vi "HEWH_Inficon.vi"(8 "error in":errorcluster, 11 "Message Queues out":T1) -> (0 "error out":errorcluster)   [LabVIEW 2023]
uses:
  Tenney/support/Message Queue/All Message Queues.ctl
  Tenney/support/Message Queue/Message Cluster.ctl
  <vilib>/NI/Modbus Library/API/Master/Modbus Master.lvclass
  Drivers/Inficon Fusion Micro GC/Type Definitions/Inficon Data.ctl
  <vilib>/NI/Modbus Library/API/Wrapper/Create TCP Master.vi
  FVIR and LDO/support/Message Queue/Enqueue Message (Single).vi
  FVIR and LDO/support/Message Queue/Message Queue.lvlib
  <vilib>/NI/Modbus Library/API/Wrapper/API Main.lvlib
  Tenney/support/Message Queue/Tenney Message Queue.lvlib
panel:
  out "Debug List":string[](array[string])
  in  "Debug":bool
  out "Loop Count":i32
  # "Need to send this value from the main program"
  # "NG Inficon: 192.168.1.32\nLP Inficon: 192.168.1.33"
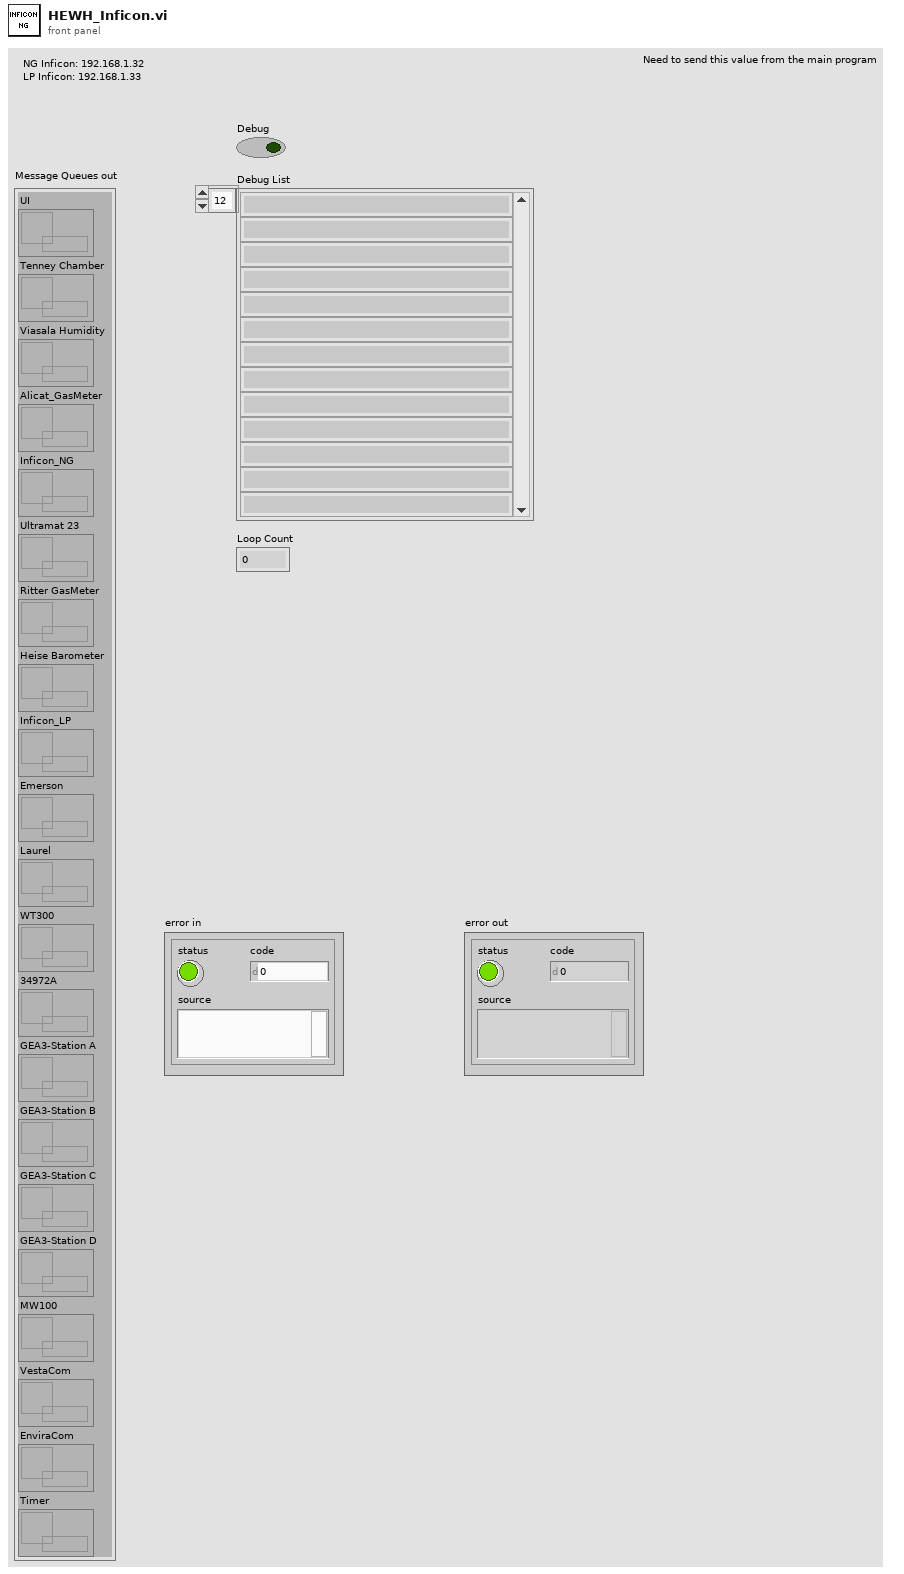
[diagram p1: front panel]
types:
  T1 = typedef "Tenney Message Queue.lvlib/All Message Queues.ctl" = cluster{"UI":refnum<queue>, "Tenney Chamber":refnum<queue>, "Viasala Humidity":refnum<queue>, "Alicat_GasMeter":refnum<queue>, "Inficon_NG":refnum<queue>, "Ultramat 23":refnum<queue>, "Ritter GasMeter":refnum<queue>, "Heise Barometer":refnum<queue>, "Inficon_LP":refnum<queue>, "Emerson":refnum<queue>, "Laurel":refnum<queue>, "WT300":refnum<queue>, "34972A":refnum<queue>, "GEA3-Station A":refnum<queue>, "GEA3-Station B":refnum<queue>, "GEA3-Station C":refnum<queue>, "GEA3-Station D":refnum<queue>, "MW100":refnum<queue>, "VestaCom":refnum<queue>, "EnviraCom":refnum<queue>, "Timer":refnum<queue>}
  T2 = typedef "Inficon Data.ctl" = cluster{"Gross Heating Value, Vol (Real, Dry)":dbl, "Nitrogen Component Normalized Mole % (Dry)":dbl, "Methane Component Normalized Mole % (Dry)":dbl, "Carbon Dioxide Component Normalized Mole % (Dry)":dbl, "Ethane Component Normalized Mole % (Dry)":dbl, "Propane Component Normalized Mole % (Dry)":dbl, "i-Pentane Component Normalized Mole % (Dry)":dbl, "i-Butane Component Normalized Mole % (Dry)":dbl, "n-Butane Component Normalized Mole % (Dry)":dbl, "n-Pentane Component Normalized Mole % (Dry)":dbl, "Hexane Component Normalized Mole % (Dry)":dbl, "Heptane Component Normalized Mole % (Dry)":dbl, "Gross Wobbe Index, Real(Dry)":dbl, "Relative Density, Real(Dry)":dbl, "Propylene Component Normalized Mole % (Dry)":dbl, "C4 Olefins Component Normalized Mole % (Dry)":dbl, "Water Component Normalized Mole % (Dry)":dbl, "Gross Heating Value, Vol (Real, Sat)":dbl, "Natural Gas Data":string[][], "Propane Data":string[][]}
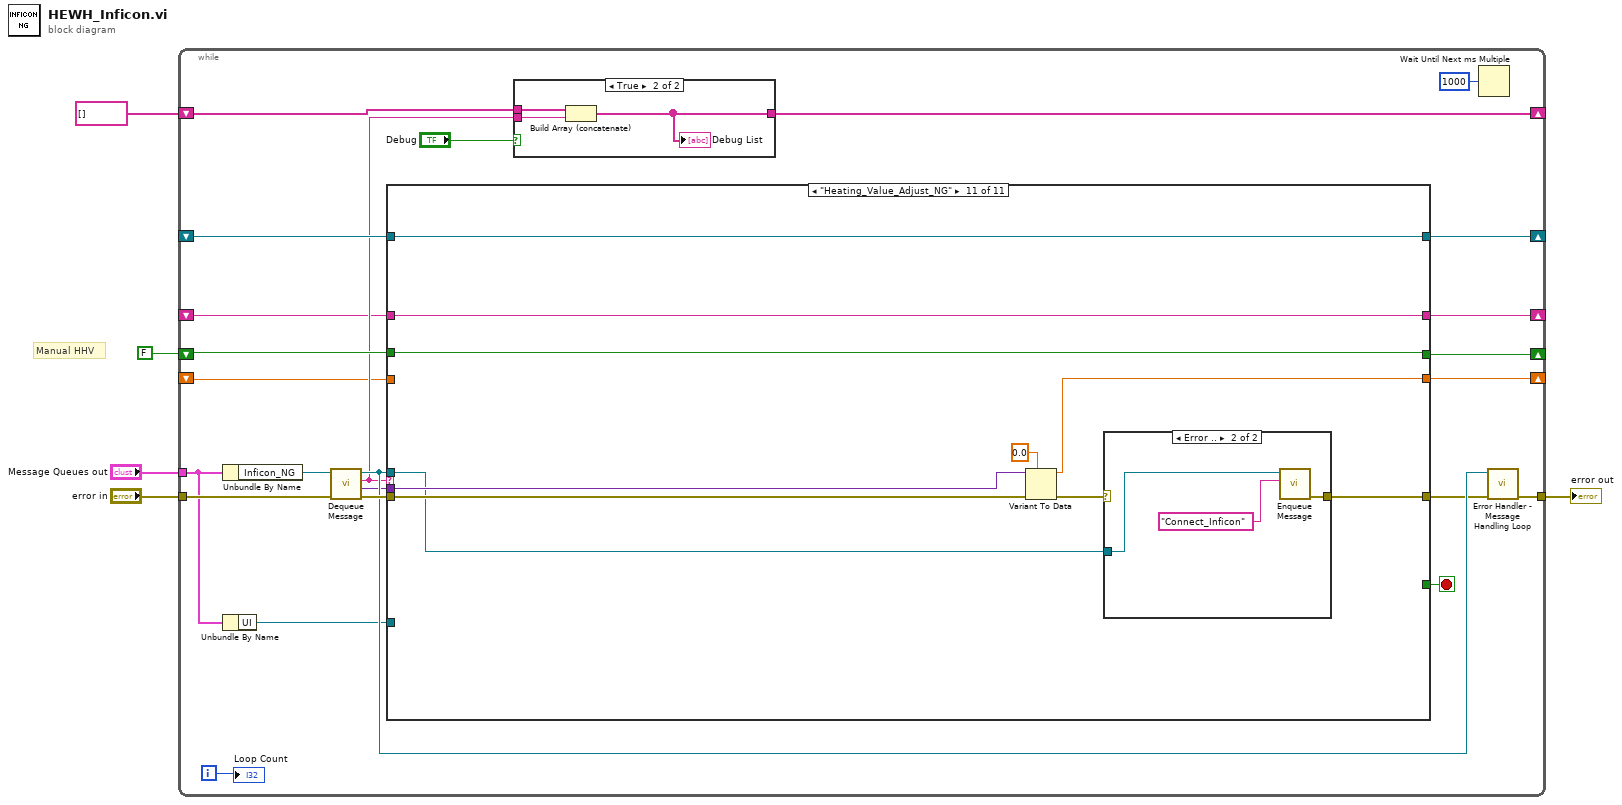
[diagram p0: block diagram]
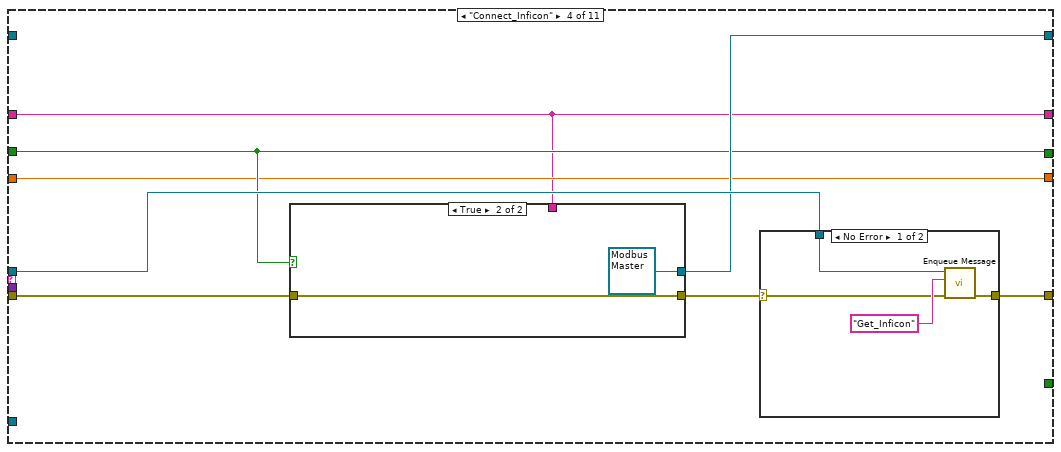
[diagram p6: hidden frame]
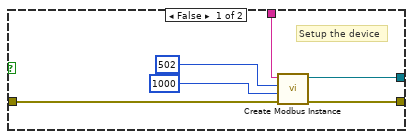
[diagram p7: hidden frame]
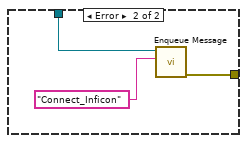
[diagram p8: hidden frame]
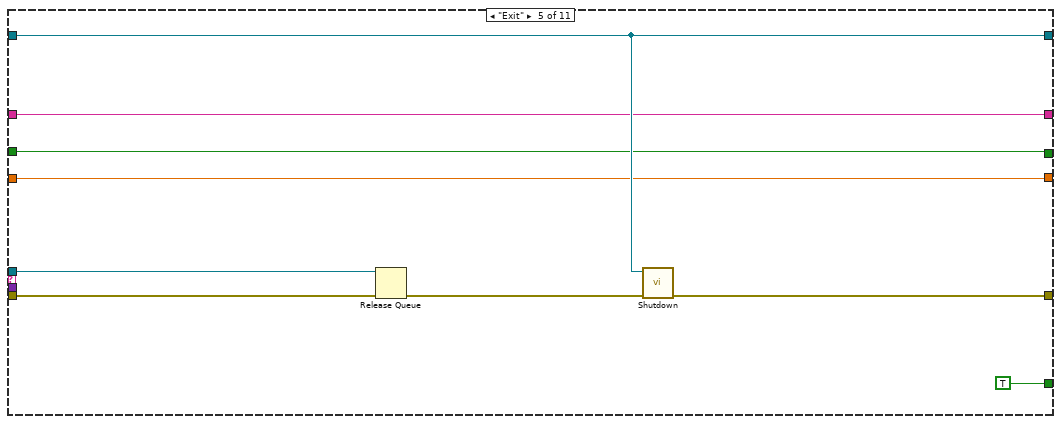
[diagram p9: hidden frame]
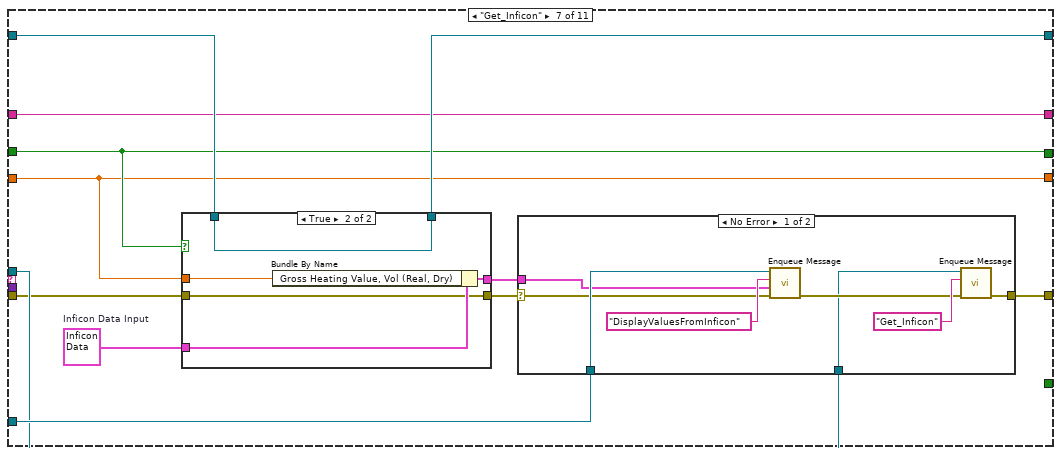
[diagram p11: hidden frame]
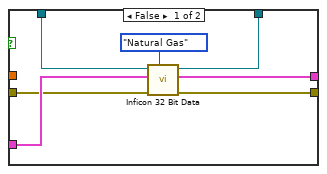
[diagram p12: hidden frame]
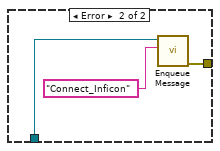
[diagram p13: hidden frame]
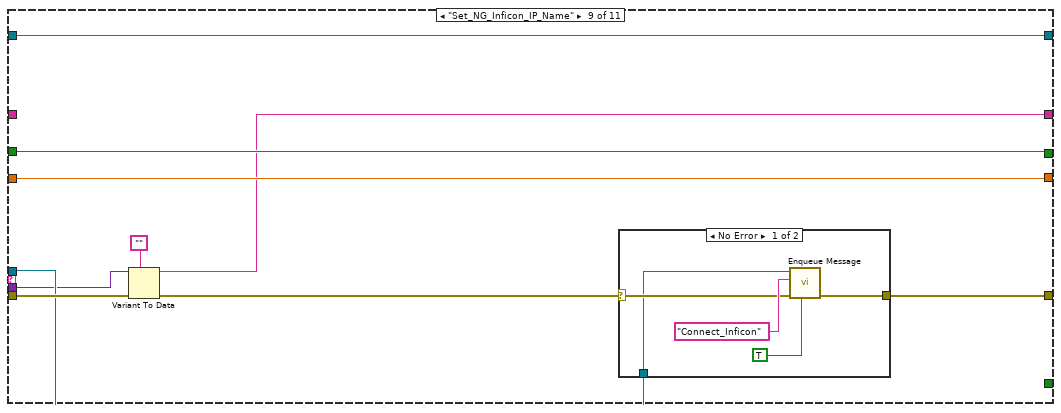
[diagram p15: hidden frame]
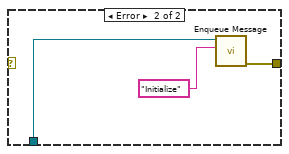
[diagram p16: hidden frame]
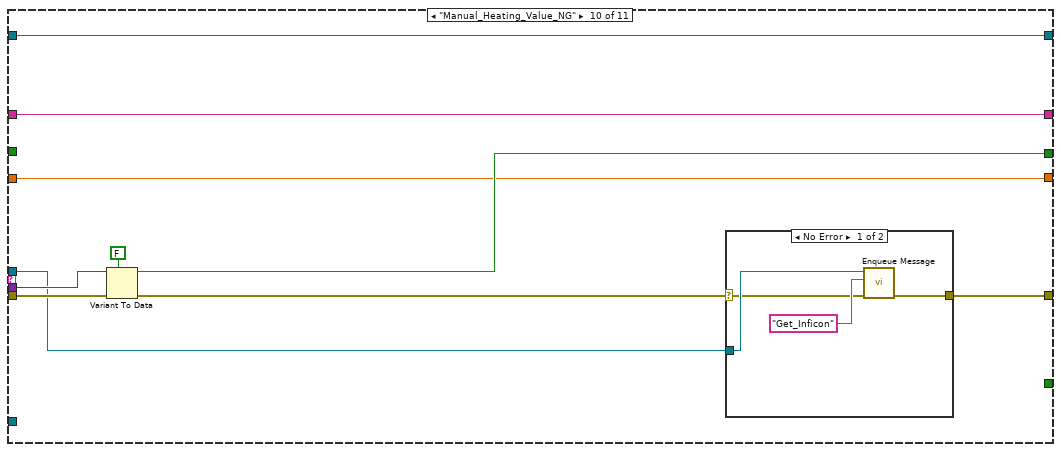
[diagram p17: hidden frame]
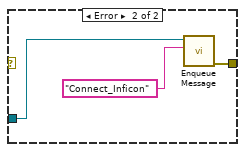
[diagram p18: hidden frame]
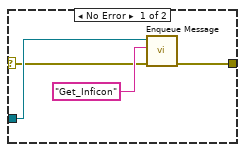
[diagram p19: hidden frame]
diagram:
  # "Manual HHV"
  n1 = while {
    tunnel: "Message Queues out" -> [w21]
    tunnel: "error in" -> [w28]
    tunnel: [w24] -> w4
    shift-right: [w19] -> _
    shift-left: _ -> [w18]
    shift-right: [w15] -> _
    shift-left: FALSE -> [w14]
    shift-right: [w10] -> _
    shift-left: string[] [] -> [w12]
    shift-right: [w9] -> _
    shift-left: _ -> [w8]
    shift-right: [w7] -> _
    shift-left: _ -> [w6]
    i -> [w17]
    stop <- w26 stop-if-true
    n2 = Unbundle By Name(w21) -> ("Inficon_NG"=w29:refnum<queue>)
    n3 = Unbundle By Name(w21) -> ("UI"=w20:refnum<queue>)
    n4 = call "Dequeue Message.vi"("error in (no error)"=w28, "Message Queue"=w29) -> ("error out"=w27:errorcluster, "Message Data"=w16:variant, "Message"=w11:string, "dup Message Queue"=w25:refnum<queue>)  [unwired: 6 in]
    n5 = case shown="\"Heating_Value_Adjust_NG\"" w11 {
      tunnel: w27 -> [w35 w40 w44 w54 w75 w82 w93 w122 w131 w152 w169]
      tunnel: [w35 w40 w44 w56 w77 w82 w96 w122 w129 w147 w166] -> w23
      tunnel: [_ _ _ _ TRUE _ _ _ _ _ _] -> w26
      tunnel: w25 -> [_ _ _ w55 w79 _ w95 _ w128 w146 w165]
      tunnel: w20 -> [_ _ _ _ _ _ w97 _ _ _ _]
      tunnel: [w38 w43 w48 w53 w76 w85 w91 w125 w135 w153 w170] -> w19
      tunnel: w18 -> [w38 w43 w48 _ w76 w85 w92 w125 w135 w153 w170]
      tunnel: w16 -> [_ _ _ _ _ _ _ _ w127 w151 w168]
      tunnel: [w37 w42 w47 w51 w74 w84 w88 w124 w134 w149 w163] -> w15
      tunnel: w14 -> [w37 w42 w47 w51 w74 w84 w88 w124 w134 _ w163]
      tunnel: [w36 w41 w46 w50 w73 w83 w87 w123 w133 w145 w162] -> w9
      tunnel: w8 -> [w36 w41 w46 w50 w73 w83 w87 w123 w133 w145 _]
      tunnel: [w34 w39 w45 w49 w72 w81 w86 w121 w126 w144 w161] -> w7
      tunnel: w6 -> [w34 w39 w45 w49 w72 w81 w86 w121 _ w144 w161]
      frame "---------- Setup ----------" {
      }
      frame Default {
      }
      frame "Initialize" {
      }
      frame "Connect_Inficon" {
        n6 = case shown="True" w51 {
          tunnel: w54 -> [w60 w64]
          tunnel: [w59 refnum<class "Modbus Master.lvclass"> refnum ("TCP master instance")] -> w53
          tunnel: [w58 w64] -> w52
          tunnel: w49 -> [w57 _]
          frame False {
            # "Setup the device"
            n7 = call-poly <vilib>:"Create Modbus Instance.vi"("error in"=w60, "connect timeout ms"=1000, "port (502)"=u16 502, "address"=w57) -> ("error out"=w58:errorcluster, "TCP master instance"=w59:refnum<class "Modbus Master.lvclass">)  [unwired: 6 in]
          }
          frame True {
          }
        }
        n8 = case shown="No Error" w52 {
          selector: w52 -> [w65 _]
          tunnel: [w67 w70] -> w56
          tunnel: w55 -> [w66 w69]
          frame No Error {
            n9 = call-poly "Enqueue Message.vi"("error in (no error)"=w65, "Message"="Get_Inficon", "Message Queue"=w66) -> ("error out"=w67:errorcluster)  [unwired: 7 in, 1 out]
          }
          frame Error {
            n10 = call-poly "Enqueue Message.vi"("Message"="Connect_Inficon", "Message Queue"=w69) -> ("error out"=w70:errorcluster)  [unwired: 8 in, 1 out]
          }
        }
      }
      frame "Exit" {
        n11 = Release Queue(queue=w79, error in (no error)=w75) -> (error out=w78:errorcluster)  [unwired: 1 in, 2 out]
        n12 = call-dynamic "Shutdown.vi"("error in"=w78, "Modbus master in"=w76) -> ("error out"=w77:errorcluster)  [unwired: 9 in]
      }
      frame "---------- Data Collection ----------" {
      }
      frame "Get_Inficon" {
        w94 = T2 {"Gross Heating Value, Vol (Real, Dry)"=0.0, "Nitrogen Component Normalized Mole % (Dry)"=0.0, "Methane Component Normalized Mole % (Dry)"=0.0, "Carbon Dioxide Component Normalized Mole % (Dry)"=0.0, "Ethane Component Normalized Mole % (Dry)"=0.0, "Propane Component Normalized Mole % (Dry)"=0.0, "i-Pentane Component Normalized Mole % (Dry)"=0.0, "i-Butane Component Normalized Mole % (Dry)"=0.0, "n-Butane Component Normalized Mole % (Dry)"=0.0, "n-Pentane Component Normalized Mole % (Dry)"=0.0, "Hexane Component Normalized Mole % (Dry)"=0.0, "Heptane Component Normalized Mole % (Dry)"=0.0, "Gross Wobbe Index, Real(Dry)"=0.0, "Relative Density, Real(Dry)"=0.0, "Propylene Component Normalized Mole % (Dry)"=0.0, "C4 Olefins Component Normalized Mole % (Dry)"=0.0, "Water Component Normalized Mole % (Dry)"=0.0, "Gross Heating Value, Vol (Real, Sat)"=0.0, "Natural Gas Data"=[], "Propane Data"=[]}  # Inficon Data Input
        n13 = case shown="True" w88 {
          tunnel: w94 -> [w104 w109]
          tunnel: w93 -> [w103 w107]
          tunnel: w92 -> [w101 w106]
          tunnel: [w100 w106] -> w91
          tunnel: [w99 w108] -> w90
          tunnel: [w98 w107] -> w89
          tunnel: w87 -> [_ w105]
          frame False {
            n14 = call "Inficon 32 Bit Data.vi"("Gas Type"=enum16{"Natural Gas", "Propane Gas"}."Natural Gas", "Error In"=w103, "Inficon Data Input"=w104, "Modbus master in"=w101) -> ("Error Out"=w98:errorcluster, "Inficon Data Output"=w99:T2, "Modbus master out"=w100:refnum<class "Modbus Master.lvclass">)  [unwired: 4 in, 1 out]
          }
          frame True {
            n15 = Bundle By Name(cluster=w109, "Gross Heating Value, Vol (Real, Dry)"=w105) -> (w108:T2)
          }
        }
        n16 = case shown="No Error" w89 {
          selector: w89 -> [w110 _]
          tunnel: w97 -> [w116 _]
          tunnel: [w113 w119] -> w96
          tunnel: w95 -> [w112 w118]
          tunnel: w90 -> [w111 _]
          frame No Error {
            n17 = call-poly "Enqueue Message.vi"("error in (no error)"=w110, "Message Data"=w111, "Message"="DisplayValuesFromInficon", "Message Queue"=w116) -> ("error out"=w114:errorcluster)  [unwired: 6 in, 1 out]
            n18 = call-poly "Enqueue Message.vi"("error in (no error)"=w114, "Message"="Get_Inficon", "Message Queue"=w112) -> ("error out"=w113:errorcluster)  [unwired: 7 in, 1 out]
          }
          frame Error {
            n19 = call-poly "Enqueue Message.vi"("Message"="Connect_Inficon", "Message Queue"=w118) -> ("error out"=w119:errorcluster)  [unwired: 8 in, 1 out]
          }
        }
      }
      frame "---------- Events ----------" {
      }
      frame "Set_NG_Inficon_IP_Name" {
        n20 = Variant To Data(error in=w131, type="", Variant=w127) -> (data=w126:string, error out=w130:errorcluster)
        n21 = case shown="No Error" w130 {
          selector: w130 -> [w138 _]
          tunnel: [w137 w142] -> w129
          tunnel: w128 -> [w136 w141]
          frame No Error {
            n22 = call-poly "Enqueue Message.vi"("Priority Message? (F)"=TRUE, "error in (no error)"=w138, "Message"="Connect_Inficon", "Message Queue"=w136) -> ("error out"=w137:errorcluster)  [unwired: 6 in, 1 out]
          }
          frame Error {
            n23 = call-poly "Enqueue Message.vi"("Message"="Initialize", "Message Queue"=w141) -> ("error out"=w142:errorcluster)  [unwired: 8 in, 1 out]
          }
        }
      }
      frame "Manual_Heating_Value_NG" {
        n24 = Variant To Data(error in=w152, type=FALSE, Variant=w151) -> (data=w149:bool, error out=w148:errorcluster)
        n25 = case shown="No Error" w148 {
          selector: w148 -> [w154 _]
          tunnel: [w156 w159] -> w147
          tunnel: w146 -> [w155 w158]
          frame No Error {
            n26 = call-poly "Enqueue Message.vi"("error in (no error)"=w154, "Message"="Get_Inficon", "Message Queue"=w155) -> ("error out"=w156:errorcluster)  [unwired: 7 in, 1 out]
          }
          frame Error {
            n27 = call-poly "Enqueue Message.vi"("Message"="Connect_Inficon", "Message Queue"=w158) -> ("error out"=w159:errorcluster)  [unwired: 8 in, 1 out]
          }
        }
      }
      frame "Heating_Value_Adjust_NG" {
        n28 = Variant To Data(error in=w169, type=0.0, Variant=w168) -> (data=w162:dbl, error out=w167:errorcluster)
        n29 = case shown="Error .." w167 {
          selector: w167 -> [w171 _]
          tunnel: [w173 w176] -> w166
          tunnel: w165 -> [w172 w175]
          frame No Error {
            n30 = call-poly "Enqueue Message.vi"("error in (no error)"=w171, "Message"="Get_Inficon", "Message Queue"=w172) -> ("error out"=w173:errorcluster)  [unwired: 7 in, 1 out]
          }
          frame Error {
            n31 = call-poly "Enqueue Message.vi"("Message"="Connect_Inficon", "Message Queue"=w175) -> ("error out"=w176:errorcluster)  [unwired: 8 in, 1 out]
          }
        }
      }
    }
    n32 = case shown="True" "Debug" {
      tunnel: w11 -> [_ w33]
      tunnel: w12 -> [w30 w32]
      tunnel: [w30 w31] -> w10
      frame False {
      }
      frame True {
        n33 = Build Array (concatenate)(w32, w33) -> (w31:string[])
        "Debug List" <- w31
      }
    }
    n34 = Wait Until Next ms Multiple(millisecond multiple=u32 1000) -> ()  [unwired: 1 out]
    n35 = call "Error Handler - Message Handling Loop.vi"("error in (no error)"=w23, "Message Queue"=w25) -> ("dup error in"=w24:errorcluster)  [unwired: 8 in, 1 out]
    "Loop Count" <- w17
  }
  "error out" <- w4
